vi "生成参数.vi"(1 "GPRS参数（TXJT）":T1={"IP地址"="000.000.000.000", "工作模式"=48, "连接协议"=48, "本机号码"="13806871122", "短信监控中心号码1"="13800577500", "监听时间"=10000, "心跳间隔"=0, "重启时间(分)"=0, "C/S关系"=49, "DNS域名"="", "APN接入点"="", "报头使能"=49, "波特率"=75, "短信目标号码1 "="", "短信目标号码2"="", "短信监控中心号码2"="", "信号检测使能"=48, "控制方式"=48, "端口号"=50700, "连接方式"=49} {"连接方式" items=["固定IP"=48, "域名解析"=49]; "控制方式" items=["软件控制"=48, "EN控制"=49]; "信号检测使能" items=["不检测"=48, "检测"=49]; "波特率" items=["1200"=45060, "2400"=24585, "4800"=49170, "9600"=32805, "19200"=75]; "报头使能" items=["上传"=48, "不上传"=49]; "C/S关系" items=["客服端"=48, "服务端"=49]; "连接协议" items=["TCP协议"=48, "UDP协议"=49]; "工作模式" items=["GPRS模式"=48, "短信模式"=49]}) -> (0 "字符串":string)   [LabVIEW 2015]
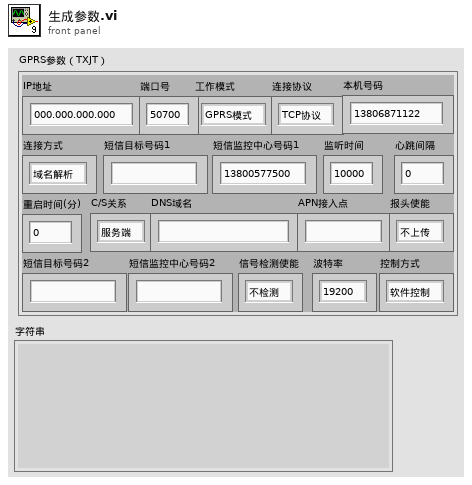
[diagram p1: front panel]
types:
  T1 = typedef "GPRS参数DW02.ctl" = cluster{"IP地址":string, "工作模式":u16, "连接协议":u16, "本机号码":string, "短信监控中心号码1":string, "监听时间":u16, "心跳间隔":u16, "重启时间(分)":u16, "C/S关系":u16, "DNS域名":string, "APN接入点":string, "报头使能":u16, "波特率":u16, "短信目标号码1 ":string, "短信目标号码2":string, "短信监控中心号码2":string, "信号检测使能":u16, "控制方式":u16, "端口号":u16, "连接方式":u16}
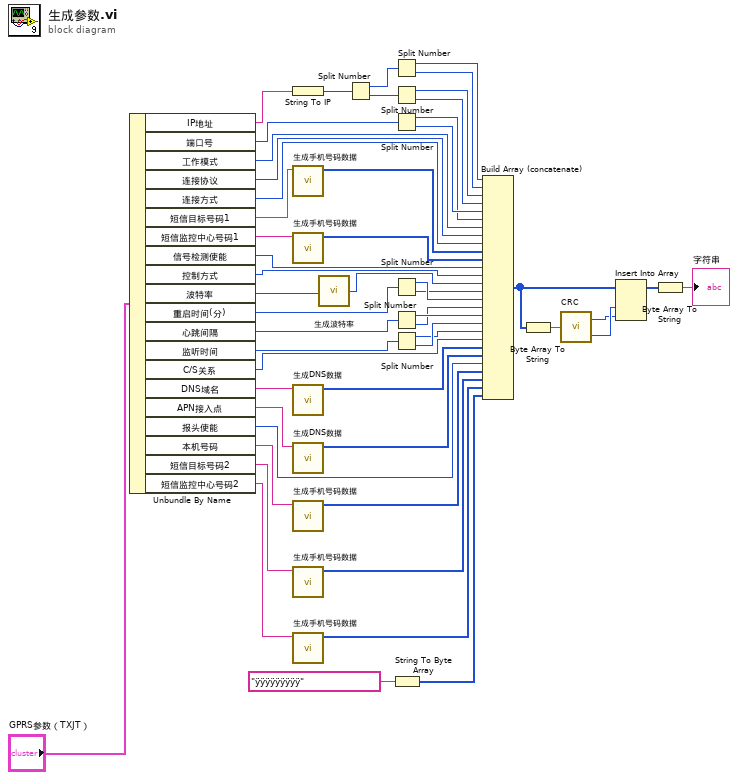
[diagram p0: block diagram]
diagram:
  n1 = Unbundle By Name("GPRS参数（TXJT）") -> ("IP地址"=w44:string, "端口号"=w43:u16, "工作模式"=w40:u16, "连接协议"=w39:u16, "连接方式"=w38:u16, "短信目标号码1"=w37:string, "短信监控中心号码1"=w35:string, "信号检测使能"=w15:u16, "控制方式"=w13:u16, "波特率"=w1:u16, "重启时间(分)"=w18:u16, "心跳间隔"=w17:u16, "监听时间"=w16:u16, "C/S关系"=w12:u16, "DNS域名"=w19:string, "APN接入点"=w27:string, "报头使能"=w11:u16, "本机号码"=w10:string, "短信目标号码2"=w24:string, "短信监控中心号码2"=w21:string)
  n2 = String To IP(1:w44) -> (0:w50:u32)
  n3 = call "生成手机号码数据.vi"("字符串"=w37) -> ("手机号码内容"=w36:u8[])  [unwired: 10 in]
  n4 = call "生成手机号码数据.vi"("字符串"=w35) -> ("手机号码内容"=w34:u8[])  [unwired: 10 in]
  n5 = call "生成DNS数据.vi"("字符串"=w19) -> ("手机号码内容"=w28:u8[])  [unwired: 10 in]
  n6 = call "生成DNS数据.vi"("字符串"=w27) -> ("手机号码内容"=w26:u8[])  [unwired: 10 in]
  n7 = call "生成手机号码数据.vi"("字符串"=w10) -> ("手机号码内容"=w25:u8[])  [unwired: 10 in]
  n8 = call "生成手机号码数据.vi"("字符串"=w24) -> ("手机号码内容"=w23:u8[])  [unwired: 10 in]
  n9 = call "生成手机号码数据.vi"("字符串"=w21) -> ("手机号码内容"=w22:u8[])  [unwired: 10 in]
  n10 = call "生成波特率.vi"("波特率"=w1) -> ("GPRS参数"=w2:i32)
  n11 = Split Number(x=w50) -> (hi(x)=w49:u16, lo(x)=w48:u16)
  n12 = Split Number(x=w49) -> (hi(x)=w20:u8, lo(x)=w47:u8)
  n13 = Split Number(x=w48) -> (hi(x)=w46:u8, lo(x)=w45:u8)
  n14 = Split Number(x=w43) -> (hi(x)=w41:u8, lo(x)=w42:u8)
  n15 = Split Number(x=w18) -> (hi(x)=w33:u8, lo(x)=w14:u8)
  n16 = Split Number(x=w17) -> (hi(x)=w32:u8, lo(x)=w31:u8)
  n17 = Split Number(x=w16) -> (hi(x)=w29:u8, lo(x)=w30:u8)
  n18 = String To Byte Array(string="ÿÿÿÿÿÿÿÿÿ" ("搜索字符串/字符(-)")) -> (unsigned byte array=w4:u8[])
  n19 = Build Array (concatenate)(w20, w47, w46, w45, w42, w41, w40, w39, w38, w36, w34, w15, w13, w2, w14, w33, w31, w32, w30, w29, w12, w28, w26, w11, w25, w23, w22, w4) -> (w8:i32[])
  n20 = Byte Array To String(unsigned byte array=w8) -> (string=w9:string)
  n21 = call "CRC.vi"("输入字符串"=w9) -> ("CRC高8位"=w6:u8, "CRC低8位"=w7:u8)
  n22 = Insert Into Array(array=w8, new element #1=w7, new element #2=w6) -> (w52:i32[])  [unwired: 1 in]
  n23 = Byte Array To String(unsigned byte array=w52) -> (string=→"字符串":string)
